vi "data update.vi"(0 "bin in":refnum<file>, 1 "sample counter in":i32, 5 "cache in":T1, 7 "data table in":T2, 9 "Time Stamp":timestamp, 11 "error in":errorcluster, 13 "scans per write":u16) -> (3 "sample counter out":i32, 4 "bin out":refnum<file>, 6 "cache out":T1, 8 "data table out":T2, 15 "error out":errorcluster)   [LabVIEW 2013, in "Binary datalogger runtime.lvclass"]
uses:
  Binary datalogger runtime.lvclass
  data cache.ctl
  <vilib>/NI/Tag Bus/table/data table.ctl
  <vilib>/NI/Tag Bus/table/data table.lvlib
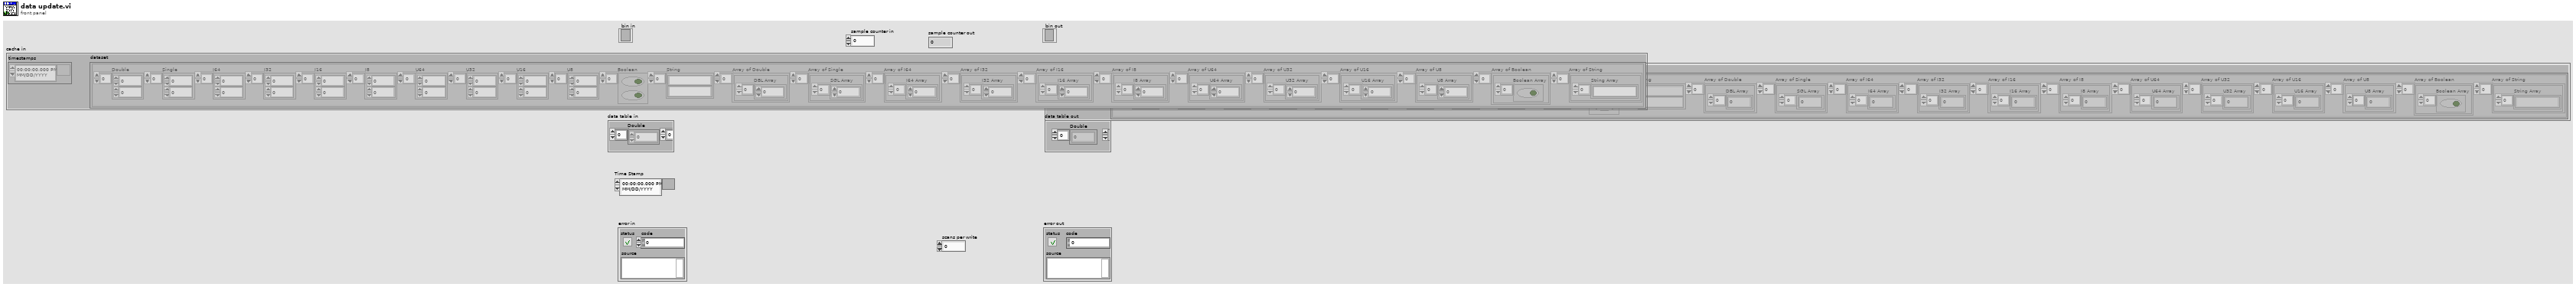
[diagram p1: front panel]
types:
  T1 = typedef "Binary datalogger runtime.lvclass/data cache.ctl" = cluster{"timestamps":timestamp[], "dataset":T2[]}
  T2 = typedef "tag bus.lvlib/data table.lvlib/data table.ctl" = cluster{"Double":dbl[], "Single":sgl[], "I64":i64[], "I32":i32[], "I16":i16[], "I8":i8[], "U64":u64[], "U32":u32[], "U16":u16[], "U8":u8[], "Boolean":bool[], "String":string[], "Array of Double":cluster{"DBL Array":dbl[]}[], "Array of Single":cluster{"SGL Array":sgl[]}[], "Array of I64":cluster{"I64 Array":i64[]}[], "Array of I32":cluster{"I32 Array":i32[]}[], "Array of I16":cluster{"I16 Array":i16[]}[], "Array of I8":cluster{"I8 Array":i8[]}[], "Array of U64":cluster{"U64 Array":u64[]}[], "Array of U32":cluster{"U32 Array":u32[]}[], "Array of U16":cluster{"U16 Array":u16[]}[], "Array of U8":cluster{"U8 Array":u8[]}[], "Array of Boolean":cluster{"Boolean Array":bool[]}[], "Array of String":cluster{"String Array":string[]}[]}
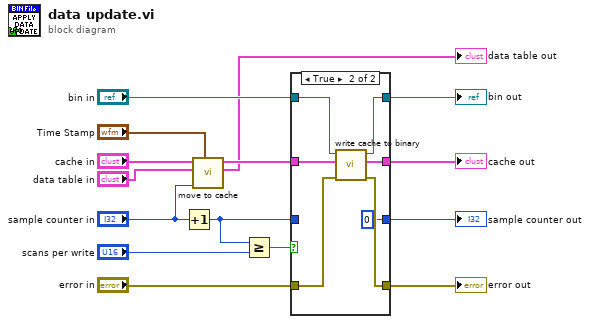
[diagram p0: block diagram]
diagram:
  n1 = Increment(x="sample counter in") -> (x+1=w15:i32)
  n2 = call "move to cache.vi"("Time Stamp"="Time Stamp", "sample counter"="sample counter in", "data table in"="data table in", "cache in"="cache in") -> ("data table out"=→"data table out":T2, "cache out"=w8:T1)  [unwired: 6 in]
  n3 = Greater Or Equal?(x=w15, y="scans per write") -> (x >= y?=w7:bool)
  n4 = case shown="True" w7 {
    tunnel: w8 -> [w19 w26]
    tunnel: [w19 w24] -> w9
    tunnel: "error in" -> [w17 w25]
    tunnel: [w17 w23] -> w11
    tunnel: [w18 w22] -> w12
    tunnel: "bin in" -> [w18 w21]
    tunnel: [w16 0] -> w14
    tunnel: w15 -> [w16 _]
    frame False {
    }
    frame True {
      n5 = call "write cache to binary.vi"("error in"=w25, "cache in"=w26, "bin file in"=w21) -> ("error out"=w23:errorcluster, "cache out"=w24:T1, "bin file out"=w22:refnum<file>)  [unwired: 6 in]
    }
  }
  "sample counter out" <- w14
  "bin out" <- w12
  "error out" <- w11
  "cache out" <- w9
